vi "Modbus Error Codes.vi"(8 "error in":errorcluster, 11 "PLC Data":T1) -> (0 "error out":errorcluster, 3 "PLC Data Output":T1)   [LabVIEW 2020, in "Modbus.lvlib"]
uses:
  Modbus.lvlib
  Modbus PLC Data All.ctl
  Modbus FVIR Control.ctl
  Modbus LDO Control.ctl
  WritingDataFile/Data to Save.ctl
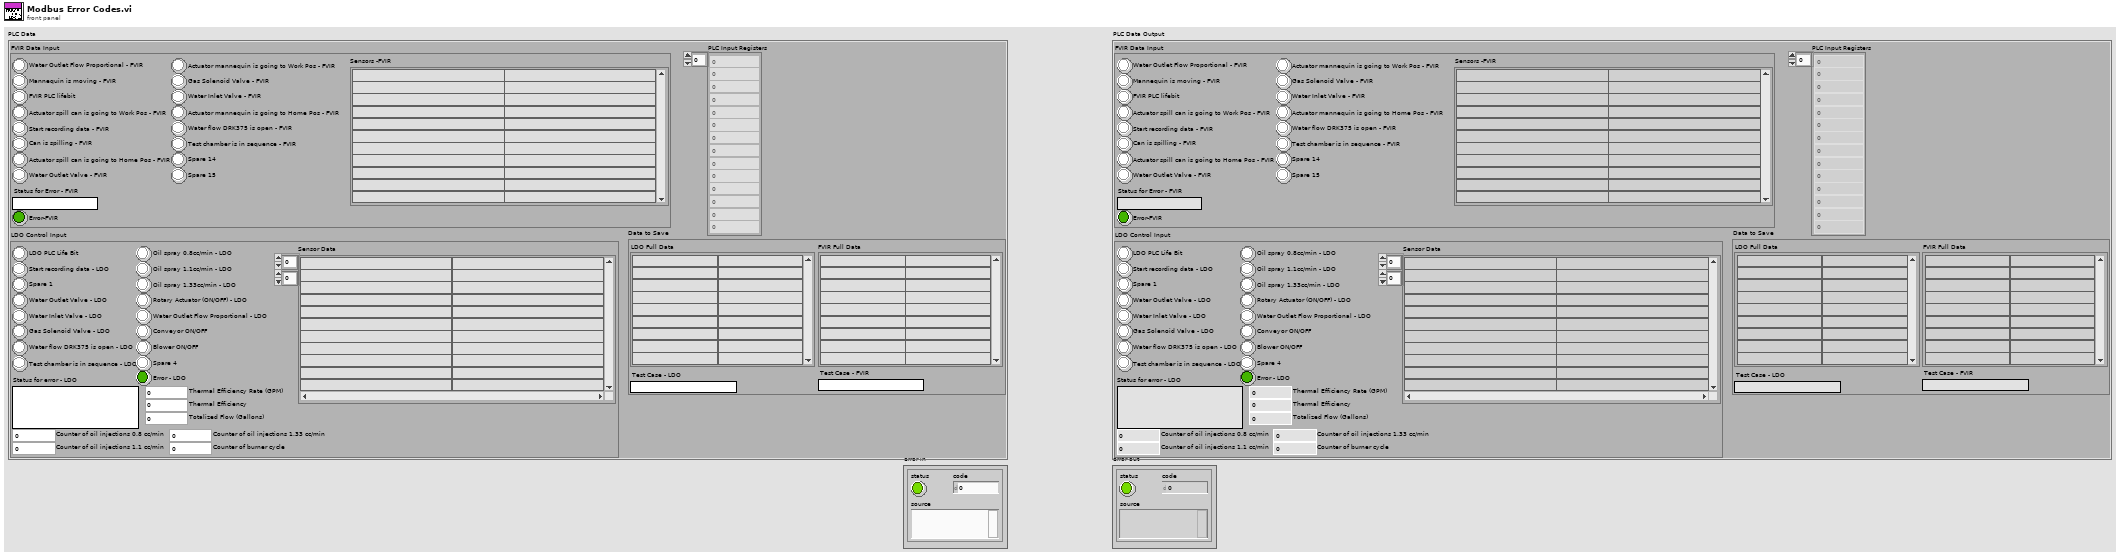
[diagram p1: front panel]
types:
  T1 = typedef "Modbus PLC Data All.ctl" = cluster{"FVIR Data Input":T2, "LDO Control Input":T3, "PLC Input Registers":i16[], "Data to Save":T4}
  T2 = typedef "Modbus FVIR Control.ctl" = cluster{"Spare 15":bool, "Spare 14":bool, "Actuator mannequin is going to Work Pos - FVIR":bool, "Actuator mannequin is going to Home Pos - FVIR":bool, "Test chamber is in sequence - FVIR ":bool, "Water flow DRK375 is open - FVIR":bool, "Gas Solenoid Valve - FVIR":bool, "Water Inlet Valve - FVIR":bool, "Water Outlet Flow Proportional - FVIR":bool, "Start recording data - FVIR":bool, "Actuator spill can is going to Work Pos - FVIR":bool, "Actuator spill can is going to Home Pos - FVIR":bool, "Water Outlet Valve - FVIR":bool, "Can is spilling - FVIR":bool, "Mannequin is moving - FVIR":bool, "FVIR PLC lifebit":bool, "Status for Error - FVIR":string, "Error-FVIR":bool, "Sensors -FVIR":string[][]}
  T3 = typedef "Modbus LDO Control.ctl" = cluster{"LDO PLC Life Bit":bool, "Start recording data - LDO":bool, "Spare 1":bool, "Water Outlet Valve - LDO":bool, "Water Inlet Valve - LDO":bool, "Gas Solenoid Valve - LDO":bool, "Water flow DRK375 is open - LDO":bool, "Test chamber is in sequence - LDO":bool, "Oil spray 0.8cc/min - LDO":bool, "Oil spray 1.1cc/min - LDO":bool, "Oil spray 1.33cc/min - LDO":bool, "Rotary Actuator (ON/OFF) - LDO":bool, "Water Outlet Flow Proportional - LDO":bool, "Conveyor ON/OFF":bool, "Blower ON/OFF":bool, "Spare 4":bool, "Status for error - LDO":string, "Error - LDO":bool, "Sensor Data":string[][], "Thermal Efficiency Rate (GPM)":dbl, "Thermal Efficiency":dbl, "Totalized Flow (Gallons)":dbl, "Counter of oil injections 1.33 cc/min":u16, "Counter of burner cycle":u16, "Counter of oil injections 1.1 cc/min":u16, "Counter of oil injections 0.8 cc/min":u16}
  T4 = typedef "Data to Save.ctl" = cluster{"LDO Full Data":string[][], "FVIR Full Data":string[][], "Test Case - FVIR":string, "Test Case - LDO":string}
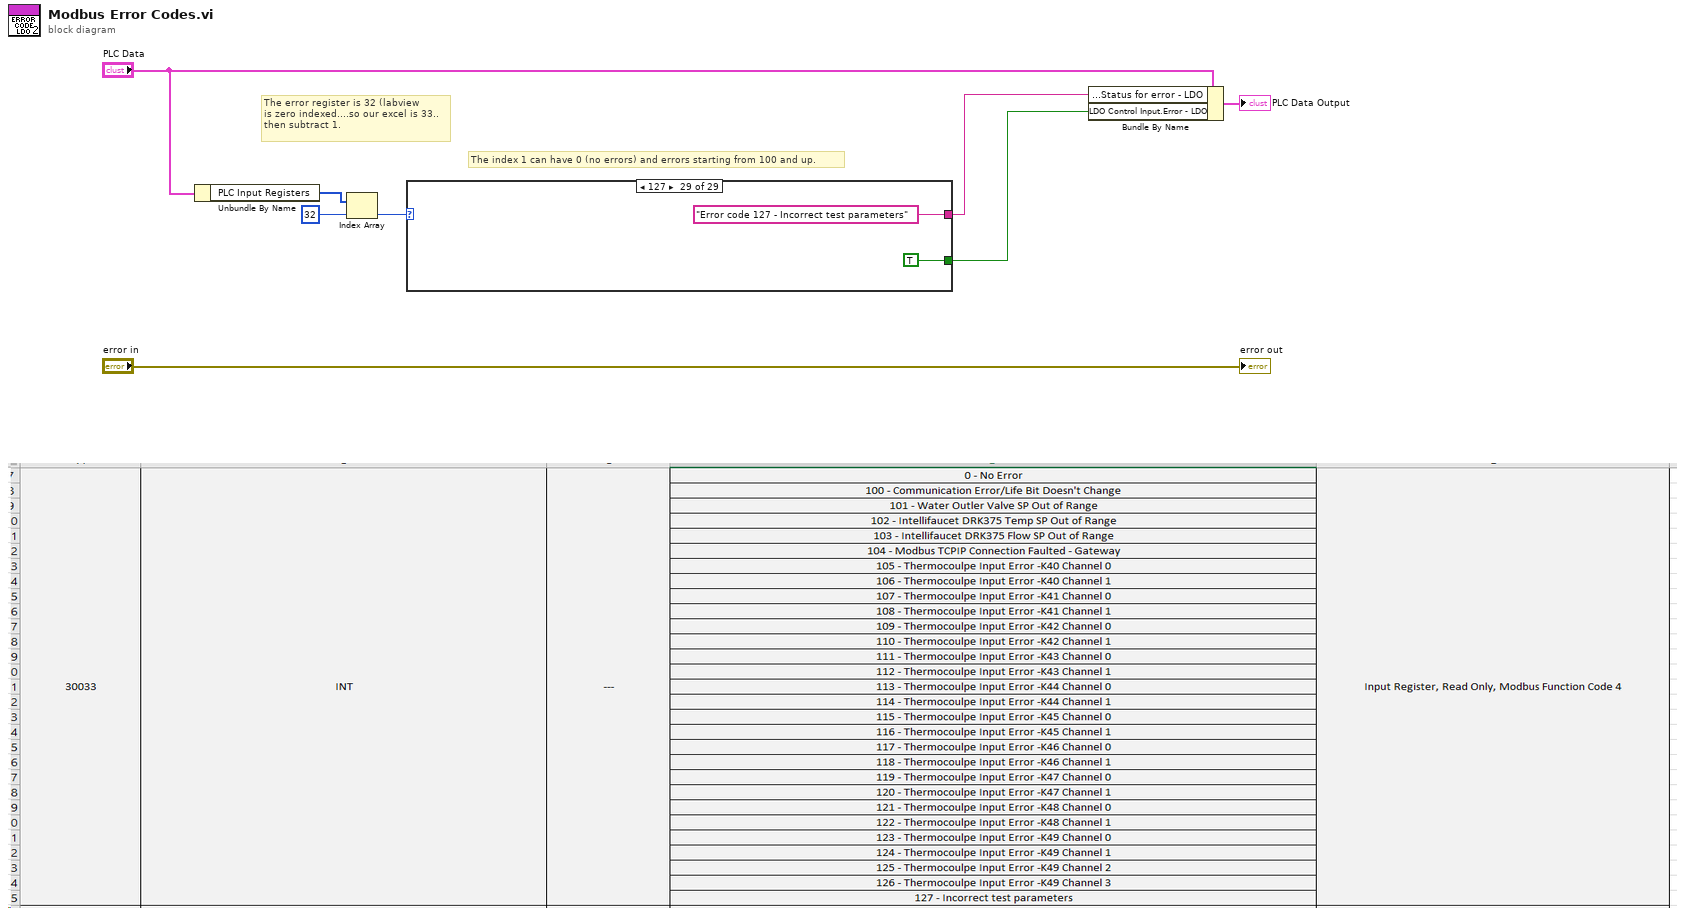
[diagram p0: block diagram]
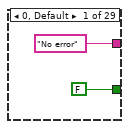
[diagram p2: hidden frame]
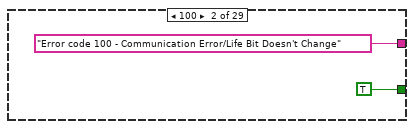
[diagram p3: hidden frame]
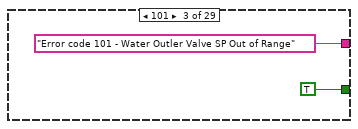
[diagram p4: hidden frame]
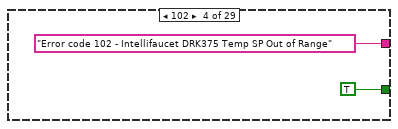
[diagram p5: hidden frame]
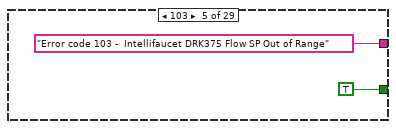
[diagram p6: hidden frame]
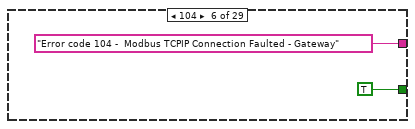
[diagram p7: hidden frame]
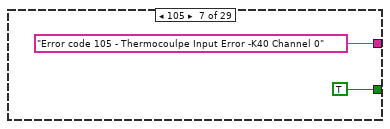
[diagram p8: hidden frame]
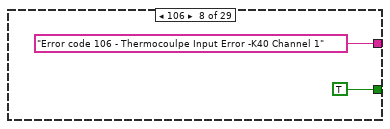
[diagram p9: hidden frame]
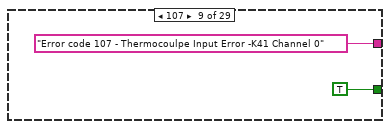
[diagram p10: hidden frame]
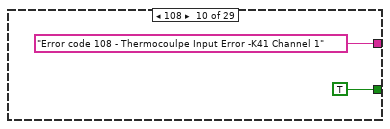
[diagram p11: hidden frame]
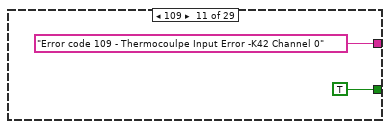
[diagram p12: hidden frame]
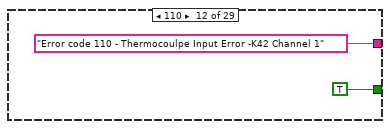
[diagram p13: hidden frame]
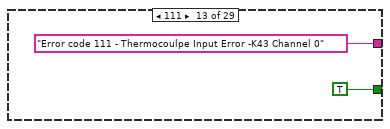
[diagram p14: hidden frame]
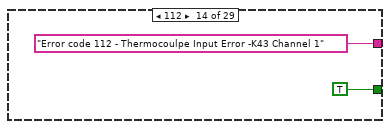
[diagram p15: hidden frame]
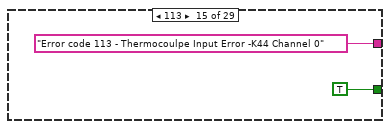
[diagram p16: hidden frame]
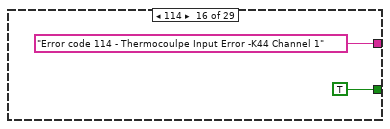
[diagram p17: hidden frame]
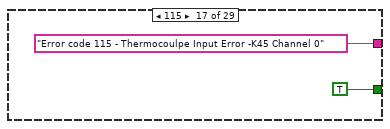
[diagram p18: hidden frame]
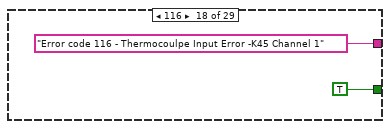
[diagram p19: hidden frame]
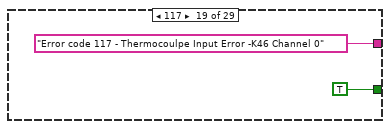
[diagram p20: hidden frame]
diagram:
  # "The error register is 32 (labview\nis zero indexed....so our excel is 33..\nthen subtract 1."
  # "The index 1 can have 0 (no errors) and errors starting from 100 and up."
  n1 = Unbundle By Name("PLC Data") -> ("PLC Input Registers"=w1:i16[])
  n2 = Index Array(array=w1, index=32) -> (element=w6:i16)
  n3 = case shown="127" w6 {
    tunnel: ["No error" "Error code 100 - Communication Error/Life Bit Doesn't Change" "Error code 101 - Water Outler Valve SP Out of Range" "Error code 102 - Intellifaucet DRK375 Temp SP Out of Range" "Error code 103 -  Intellifaucet DRK375 Flow SP Out of Range" "Error code 104 -  Modbus TCPIP Connection Faulted - Gateway" "Error code 105 - Thermocoulpe Input Error -K40 Channel 0" "Error code 106 - Thermocoulpe Input Error -K40 Channel 1" "Error code 107 - Thermocoulpe Input Error -K41 Channel 0" "Error code 108 - Thermocoulpe Input Error -K41 Channel 1" "Error code 109 - Thermocoulpe Input Error -K42 Channel 0" "Error code 110 - Thermocoulpe Input Error -K42 Channel 1" "Error code 111 - Thermocoulpe Input Error -K43 Channel 0" "Error code 112 - Thermocoulpe Input Error -K43 Channel 1" "Error code 113 - Thermocoulpe Input Error -K44 Channel 0" "Error code 114 - Thermocoulpe Input Error -K44 Channel 1" "Error code 115 - Thermocoulpe Input Error -K45 Channel 0" "Error code 116 - Thermocoulpe Input Error -K45 Channel 1" "Error code 117 - Thermocoulpe Input Error -K46 Channel 0" "Error code 118 - Thermocoulpe Input Error -K46 Channel 1" "Error code 119 - Thermocoulpe Input Error -K47 Channel 0" "Error code 120 - Thermocoulpe Input Error -K47 Channel 1" "Error code 121 - Thermocoulpe Input Error -K48 Channel 0" "Error code 122 - Thermocoulpe Input Error -K48 Channel 1" "Error code 123 - Thermocoulpe Input Error -K49 Channel 0" "Error code 124 - Thermocoulpe Input Error -K49 Channel 1" "Error code 125 - Thermocoulpe Input Error -K49 Channel 2" "Error code 126 - Thermocoulpe Input Error -K49 Channel 3" "Error code 127 - Incorrect test parameters"] -> w5
    tunnel: [FALSE TRUE TRUE TRUE TRUE TRUE TRUE TRUE TRUE TRUE TRUE TRUE TRUE TRUE TRUE TRUE TRUE TRUE TRUE TRUE TRUE TRUE TRUE TRUE TRUE TRUE TRUE TRUE TRUE] -> w4
    frame 0, Default {
    }
    frame 100 {
    }
    frame 101 {
    }
    frame 102 {
    }
    frame 103 {
    }
    frame 104 {
    }
    frame 105 {
    }
    frame 106 {
    }
    frame 107 {
    }
    frame 108 {
    }
    frame 109 {
    }
    frame 110 {
    }
    frame 111 {
    }
    frame 112 {
    }
    frame 113 {
    }
    frame 114 {
    }
    frame 115 {
    }
    frame 116 {
    }
    frame 117 {
    }
    frame 118 {
    }
    frame 119 {
    }
    frame 120 {
    }
    frame 121 {
    }
    frame 122 {
    }
    frame 123 {
    }
    frame 124 {
    }
    frame 125 {
    }
    frame 126 {
    }
    frame 127 {
    }
  }
  n4 = Bundle By Name(cluster="PLC Data", "LDO Control Input.Status for error - LDO"=w5, "LDO Control Input.Error - LDO"=w4) -> (→"PLC Data Output":T1)
  "error out" <- "error in"
